vi "19_RS232_COVID_19.vi"() -> ()   [LabVIEW 2019]
uses:
  <vilib>/Instr/_visa.llb/VISA Configure Serial Port (Instr).vi
panel:
  out "return count":u32
  out "VISA resource name out":refnum<visa-resource-name>
  in  "flow control (0:none)":u16(ring) items=["None", "XON/XOFF", "RTS/CTS", "XON/XOFF & RTS/CTS", "DTR/DSR", "XON/XOFF & DTR/DSR"]
  in  "stop bits (10: 1 bit)":u16(ring)=10 items=["1.0"=10, "1.5"=15, "2.0"=20]
  in  "error in (no error)":errorcluster
  in  "parity (0:none)":enum16{"None", "Odd", "Even", "Mark", "Space"}(ring)
  in  "data bits (8)":u16=8 min=5 max=8 step=1
  in  "baud rate (9600)":u32=9600
  in  "Enable Termination\nChar (T)":bool
  in  "termination char\n(0xA = '\\n' = LF)":u8=10 format="%.0x"
  in  "timeout (10sec)":u32=10000
  in  "VISA resource name":refnum<visa-resource-name>
  in  "BUFFER_WRITE":string
  in  "ESCRIBIR":bool
  in  "leer":bool
  out "BUFFER_READ":string
  in  "stop":bool
  # "PLANTILLA TELEMÁTICA"
  # "(C) 2020"
  # "J.LUIS PÉREZ DEL VAL"
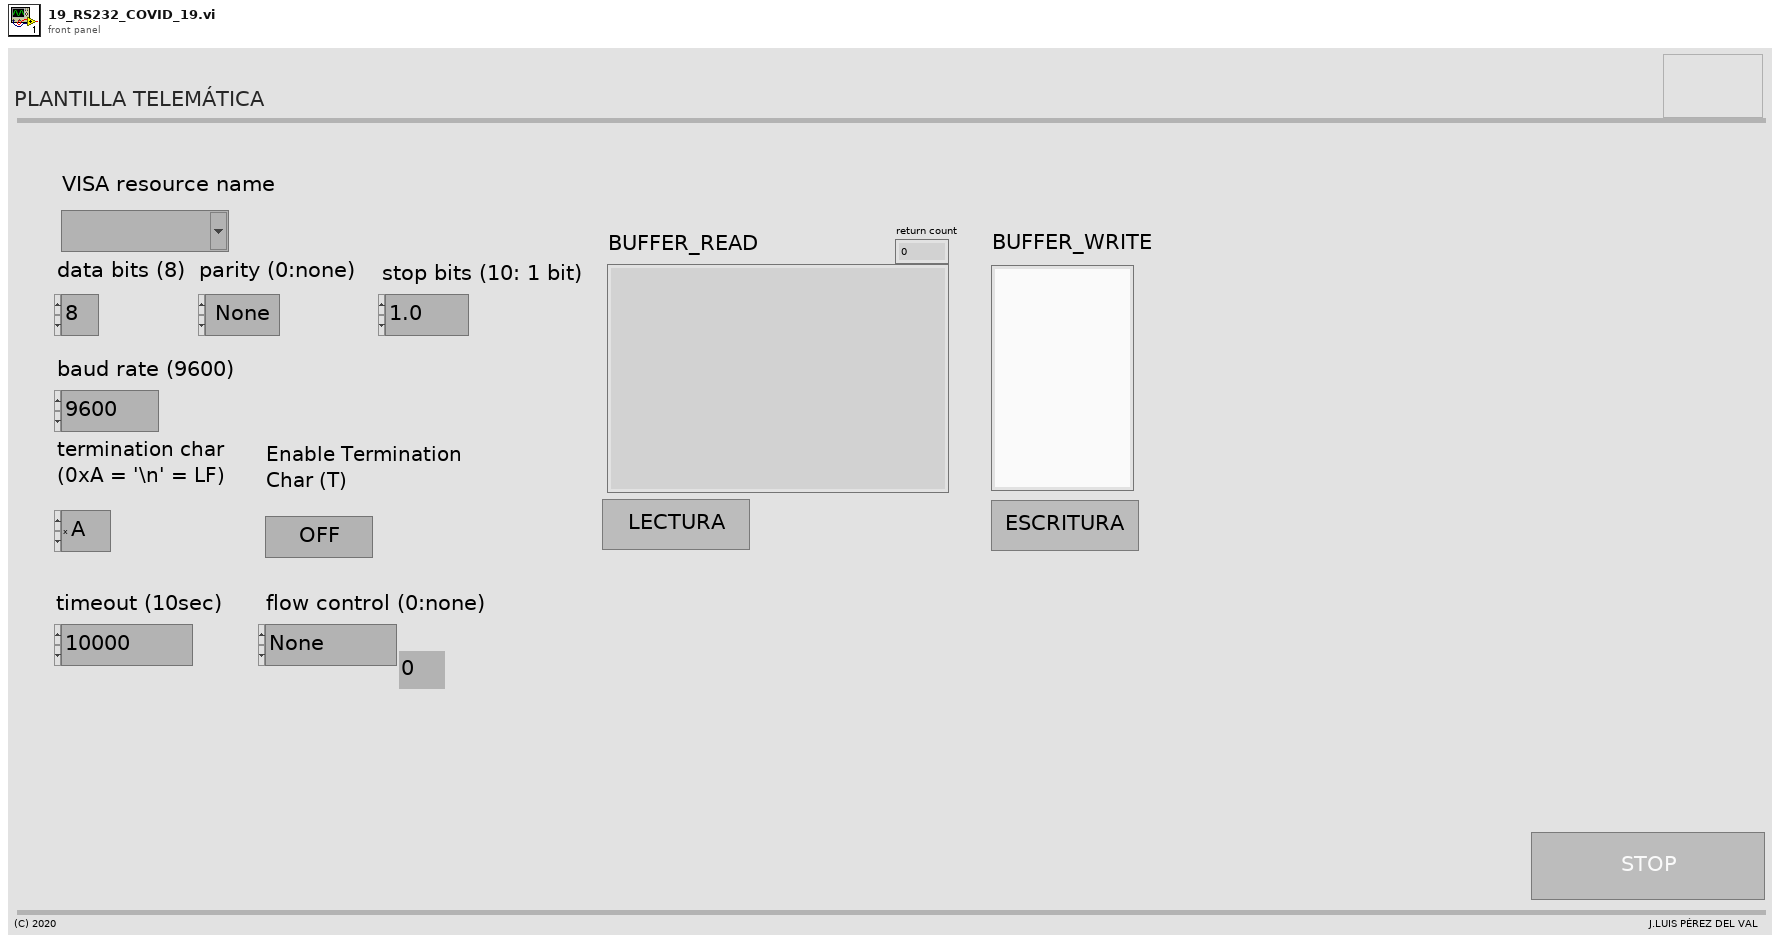
[diagram p1: front panel]
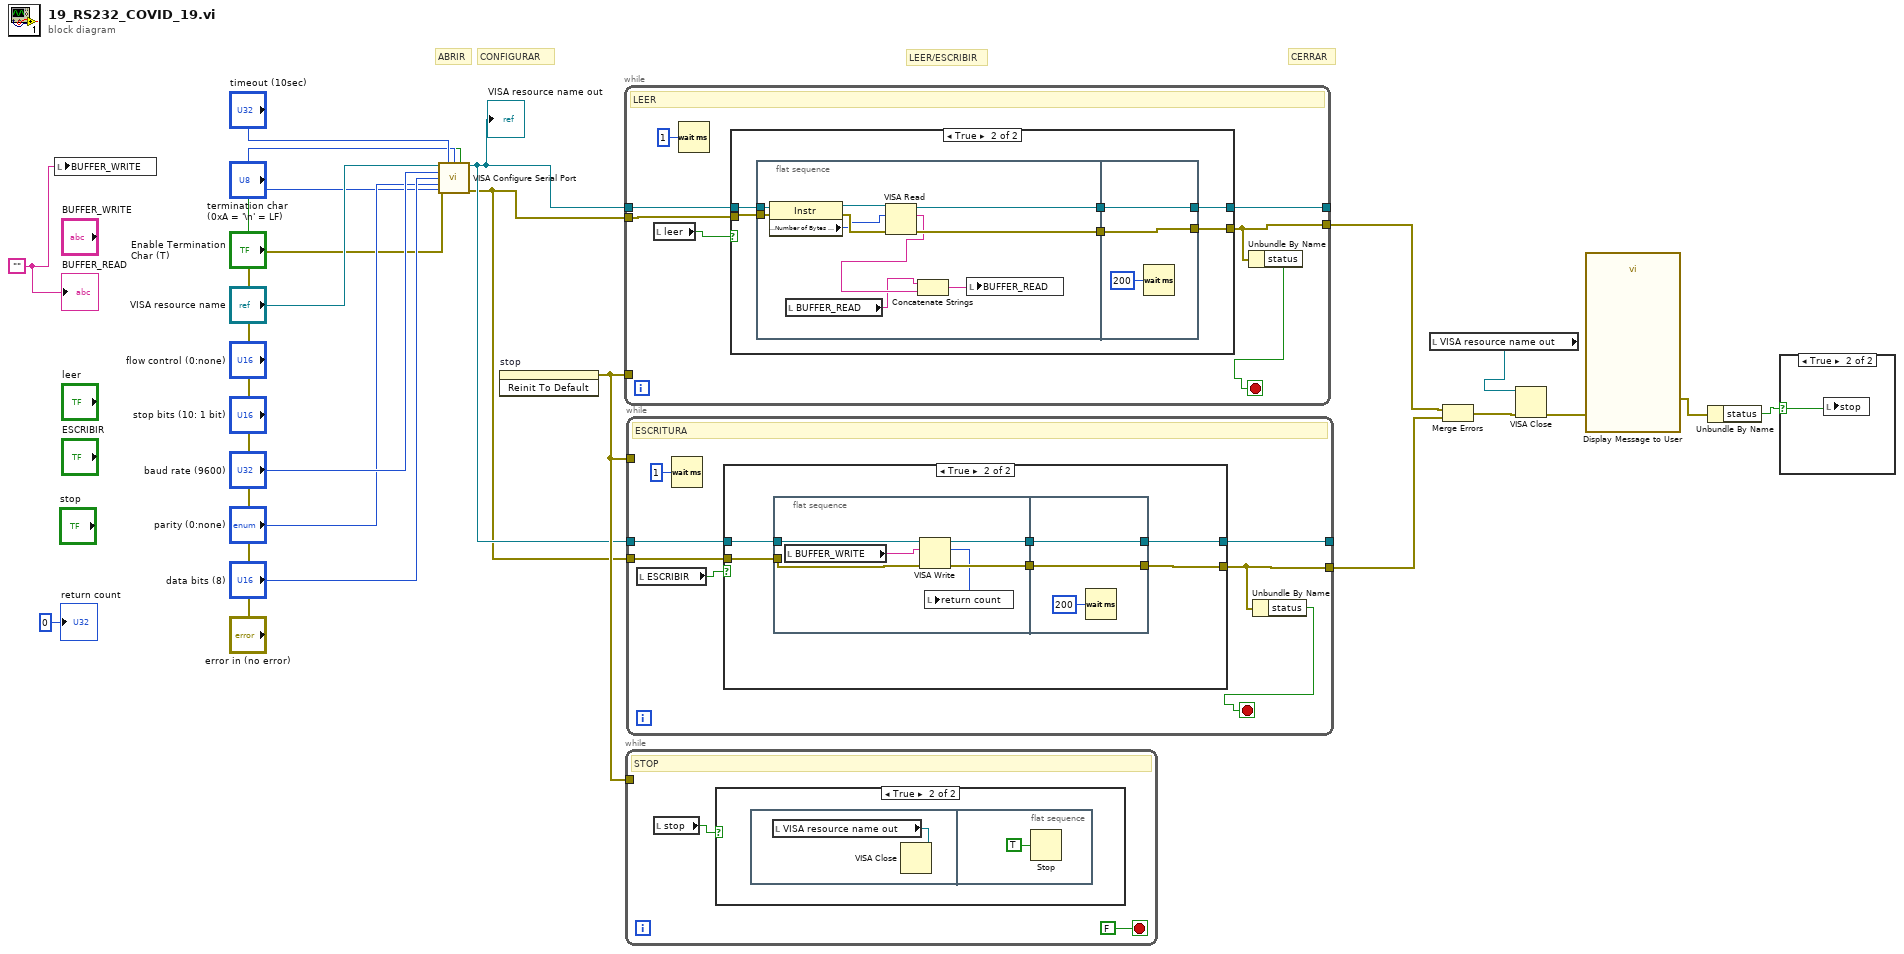
[diagram p0: block diagram]
diagram:
  w11 = ""
  # "CERRAR"
  # "LEER/ESCRIBIR"
  # "CONFIGURAR"
  # "ABRIR"
  n1 = local write "BUFFER_WRITE"(w11) -> ()
  n2 = call-poly "VISA Configure Serial Port"("VISA resource name"="VISA resource name", "timeout (10sec)"="timeout (10sec)", "termination char\n(0xA = '\\n' = LF)"="termination char\n(0xA = '\\n' = LF)", "Enable Termination\nChar (T)"="Enable Termination\nChar (T)", "baud rate (9600)"="baud rate (9600)", "data bits (8)"="data bits (8)", "parity (0:none)"="parity (0:none)", "error in (no error)"="error in (no error)", "stop bits (10: 1 bit)"="stop bits (10: 1 bit)", "flow control (0:none)"="flow control (0:none)") -> ("VISA resource name out"=w10:refnum<visa-resource-name>, "error out"=w9:errorcluster)  [unwired: 4 in]
  "VISA resource name out" <- w10
  n3 = invoke on="stop" class="Bool (strict)" method="Reinit To Default"() -> (error out=w12:errorcluster)  [unwired: 3 in, 2 out]
  n4 = while {
    tunnel: w12 -> [_]
    tunnel: w10 -> [w27]
    tunnel: w9 -> [w26]
    tunnel: [w25] -> _
    tunnel: [w24] -> w5
    stop <- w23 stop-if-true
    # "LEER"
    n5 = local read "leer"() -> (w28:bool)
    n6 = Wait (ms)(milliseconds to wait=u32 1) -> ()  [unwired: 1 out]
    n7 = case shown="True" w28 {
      tunnel: w27 -> [w31 w37]
      tunnel: w26 -> [w30 w36]
      tunnel: [w31 w34] -> w25
      tunnel: [w30 w33] -> w24
      frame False {
      }
      frame True {
        n8 = flat-sequence {
          tunnel: w37 -> [w47]
          tunnel: w36 -> [w45]
          tunnel: [w42] -> w35
          tunnel: [w41] -> w32
          tunnel: [w49] -> w34
          tunnel: w35 -> [w49]
          tunnel: [w48] -> w33
          tunnel: w32 -> [w48]
          frame #0 {
            n9 = property class="Instr"(reference=w47, error in=w45) -> (reference out=w46:refnum<visa-resource-name>, error out=w44:errorcluster, "Serial Settings:Number of Bytes at Serial Port"=w43:u32)
            n10 = local read "BUFFER_READ"() -> (w38:string)
            n11 = VISA Read(VISA resource name=w46, byte count=w43, error in (no error)=w44) -> (VISA resource name out=w42:refnum<visa-resource-name>, read buffer=w40:string, error out=w41:errorcluster)  [unwired: 1 out]
            n12 = Concatenate Strings(w38, w40) -> (w39:string)
            n13 = local write "BUFFER_READ"(w39) -> ()
          }
          frame #1 {
            n14 = Wait (ms)(milliseconds to wait=u32 200) -> ()  [unwired: 1 out]
          }
        }
      }
    }
    n15 = Unbundle By Name(w24) -> ("status"=w23:bool)
  }
  n16 = while {
    tunnel: w12 -> [_]
    stop <- FALSE stop-if-true
    # "STOP"
    n17 = local read "stop"() -> (w51:bool)
    n18 = case shown="True" w51 {
      frame False {
      }
      frame True {
        n19 = flat-sequence {
          frame #0 {
            n20 = local read "VISA resource name out"() -> (w53:refnum<visa-resource-name>)
            n21 = VISA Close(VISA resource name=w53) -> ()  [unwired: 1 in, 1 out]
          }
          frame #1 {
            n22 = Stop(stop? (T)=TRUE) -> ()
          }
        }
      }
    }
  }
  n23 = while {
    tunnel: w12 -> [_]
    tunnel: w10 -> [w59]
    tunnel: w9 -> [w58]
    tunnel: [w57] -> _
    tunnel: [w56] -> w6
    stop <- w55 stop-if-true
    # "ESCRITURA"
    n24 = local read "ESCRIBIR"() -> (w60:bool)
    n25 = Wait (ms)(milliseconds to wait=u32 1) -> ()  [unwired: 1 out]
    n26 = case shown="True" w60 {
      tunnel: w59 -> [w63 w69]
      tunnel: w58 -> [w62 w68]
      tunnel: [w63 w67] -> w57
      tunnel: [w62 w65] -> w56
      frame False {
      }
      frame True {
        n27 = flat-sequence {
          tunnel: w69 -> [w75]
          tunnel: w68 -> [w74]
          tunnel: [w72] -> w66
          tunnel: [w71] -> w64
          tunnel: [w77] -> w67
          tunnel: w66 -> [w77]
          tunnel: [w76] -> w65
          tunnel: w64 -> [w76]
          frame #0 {
            n28 = local read "BUFFER_WRITE"() -> (w73:string)
            n29 = VISA Write(VISA resource name=w75, write buffer=w73, error in (no error)=w74) -> (VISA resource name out=w72:refnum<visa-resource-name>, return count=w70:u32, error out=w71:errorcluster)
            n30 = local write "return count"(w70) -> ()
          }
          frame #1 {
            n31 = Wait (ms)(milliseconds to wait=u32 200) -> ()  [unwired: 1 out]
          }
        }
      }
    }
    n32 = Unbundle By Name(w56) -> ("status"=w55:bool)
  }
  n33 = local read "VISA resource name out"() -> (w4:refnum<visa-resource-name>)
  n34 = Merge Errors(w5, w6) -> (w7:errorcluster)
  n35 = VISA Close(VISA resource name=w4, error in (no error)=w7) -> (error out=w2:errorcluster)
  n36 = call "Display Message to User"("error in (no error)"=w2) -> ("error out"=w1:errorcluster)  [unwired: 9 in, 1 out]
  n37 = Unbundle By Name(w1) -> ("status"=w3:bool)
  n38 = case shown="True" w3 {
    selector: w3 -> [_ w79]
    frame False {
    }
    frame True {
      n39 = local write "stop"(w79) -> ()
    }
  }
  "BUFFER_READ" <- w11
  "return count" <- u32 0 ("return count")
